vi "frequency.vi"() -> ()   [LabVIEW 2014]
uses:
  <vilib>/measure/NI_MABase.lvlib
panel:
  out "Frequency 2":waveform(dbl)(graph) caption="Frequency"
  in  "stop":bool
  out "Frequency":dbl
  in  "amplitude":dbl=1.0 format="%0.2p"
  in  "frequency":dbl=10.0 format="%0.2p"
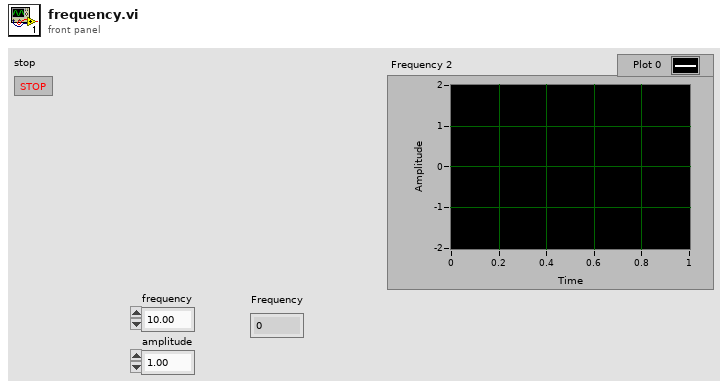
[diagram p1: front panel]
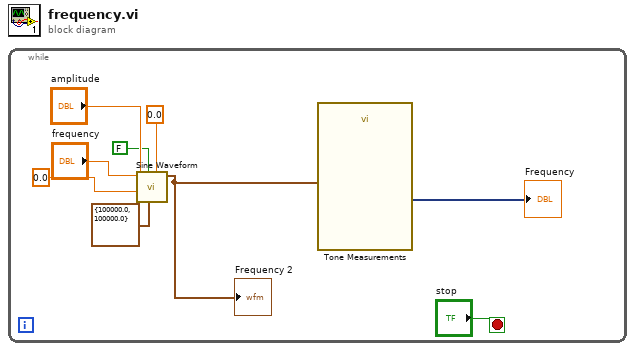
[diagram p0: block diagram]
diagram:
  n1 = while {
    stop <- "stop" stop-if-true
    n2 = call <vilib>:"Sine Waveform.vi"("offset"=0.0, "sampling info"=cluster{"Fs":dbl, "#s":dbl} {"Fs"=100000.0, "#s"=100000.0}, "reset signal"=FALSE, "phase"=0.0, "amplitude"="amplitude", "frequency"="frequency") -> ("signal out"=w1:waveform(dbl))  [unwired: 4 in, 1 out]
    "Frequency 2" <- w1
    n3 = call "Tone Measurements"("Signals"=w1) -> ("Frequency"=→"Frequency":dynamicdata)  [unwired: 9 in, 1 out]
  }
